vi "LXMCU_40G.vi"(8 "error in (no error)":errorcluster caption="错误输入（无错误）", 9 "array input":bool[][](array[boolean]), 10 "VISA COM":refnum<visa-resource-name>="COM3", 11 "LXMCU_40G输入":refnum<class "LXMCU_40G.lvclass">) -> (0 "error out":errorcluster caption="错误输出", 3 "LXMCU_40G输出":refnum<class "LXMCU_40G.lvclass">)   [LabVIEW 2011, in "LXMCU_40G.lvclass"]
uses:
  LXMCU_40G.lvclass
  LXMCU_40G.lvclass/LXMCU_40G.ctl
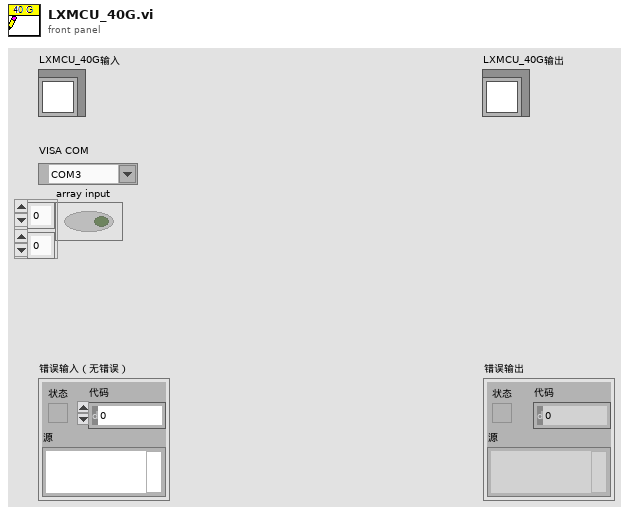
[diagram p1: front panel]
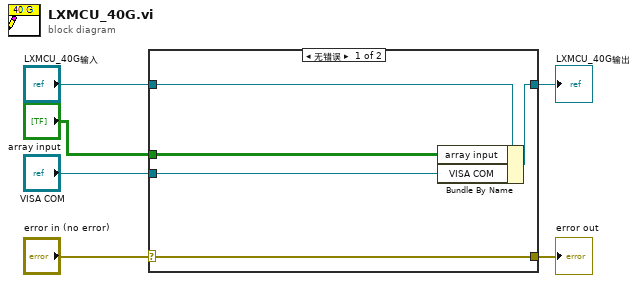
[diagram p0: block diagram]
diagram:
  n1 = case shown="无错误" "error in (no error)" {
    selector: "error in (no error)" -> [w11 w12]
    tunnel: [w11 w12] -> w5
    tunnel: [w9 w13] -> w3
    tunnel: "LXMCU_40G输入" -> [w10 w13]
    tunnel: "VISA COM" -> [w8 _]
    tunnel: "array input" -> [w7 _]
    frame No Error {
      n2 = Bundle By Name(cluster=w10, "array input"=w7, "VISA COM"=w8) -> (w9:refnum<class "LXMCU_40G.lvclass">)
    }
    frame Error {
    }
  }
  "error out" <- w5
  "LXMCU_40G输出" <- w3
